vi "Eval LTFC.vi"(8 "error in (no error)":errorcluster, 10 "Desired Field (T)":dbl) -> (0 "error out":errorcluster, 2 "Desired Control Voltage":dbl)   [LabVIEW 2009, in "Varian Magnet.lvclass"]
doc: "Evaluates Long-Term Field Calibration for control voltage that corresponds to desired field.\nAlso error checks to see if Long-Term Field Calibration is initialized properly."
uses:
  Varian Magnet.lvclass
  Varian Constants.vi
  <vilib>/Utility/error.llb/DialogType.ctl
  <vilib>/gmath/NI_Gmath.lvlib
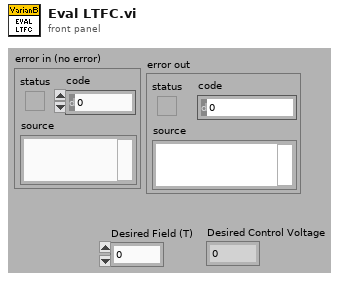
[diagram p1: front panel]
types:
  T1 = typedef "NI_Gmath.lvlib/in_piecewise interp poly control.ctl" = cluster{"x locations":dbl[], "coefficients":dbl[][]}
  T2 = typedef "DialogType.ctl" = u16
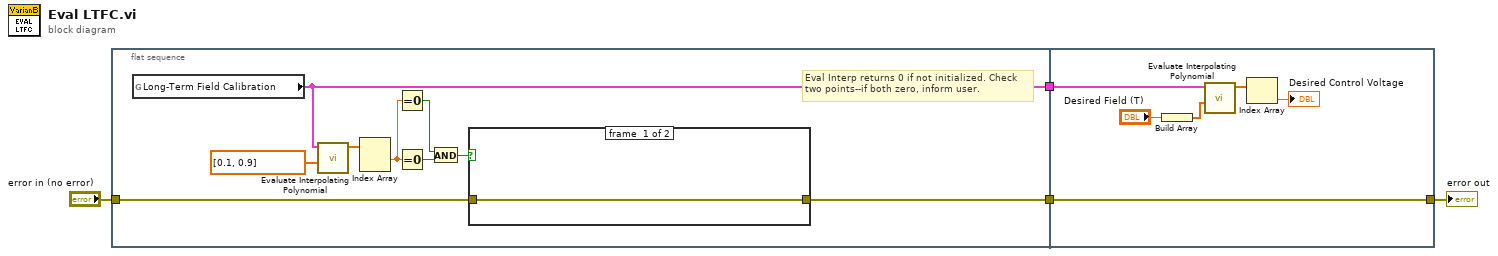
[diagram p0: block diagram]
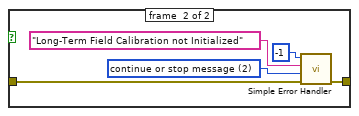
[diagram p2: hidden frame]
diagram:
  n1 = flat-sequence {
    tunnel: "error in (no error)" -> [w7]
    tunnel: [w6] -> w3
    tunnel: [w5] -> w2
    tunnel: [w25] -> w1
    tunnel: w3 -> [w25]
    tunnel: w2 -> [w23]
    frame #0 {
      # "Eval Interp returns 0 if not initialized. Check\ntwo points--if both zero, inform user."
      n2 = global read "Varian Constants.vi" "Long-Term Field Calibration"() -> (w5:T1)
      n3 = call <vilib>:"Evaluate Interpolating Polynomial.vi"("xi"=dbl[] [0.1, 0.9], "piecewise polynomial"=w5) -> ("yi"=w13:dbl[])  [unwired: 8 in, 1 out]
      n4 = Index Array(array=w13) -> (element #1=w11:dbl)  [unwired: 2 in, 1 out]
      n5 = Equal To 0?(x=w11) -> (x = 0?=w10:bool)
      n6 = Equal To 0?(x=w11) -> (x = 0?=w9:bool)
      n7 = And(x=w10, y=w9) -> (x .and. y?=w8:bool)
      n8 = case shown="True" w8 {
        tunnel: w7 -> [w14 w16]
        tunnel: [w14 w15] -> w6
        frame #0 {
        }
        frame #1 {
          w17 = T2 2 items=["no dialog", "OK message", "continue or stop message", "OK message + warnings", "continue/stop + warnings"] ("type of dialog (OK msg:1)")
          n9 = call <vilib>:"Simple Error Handler.vi"("error code (no error:0)"=-1, "error source (\" \")"="Long-Term Field Calibration not Initialized" ("error source (\" \")"), "type of dialog (OK msg:1)"=w17, "error in (no error)"=w16) -> ("error out"=w15:errorcluster)  [unwired: 1 in, 4 out]
        }
      }
    }
    frame #1 {
      n10 = Build Array("Desired Field (T)") -> (w21:dbl[])
      n11 = call <vilib>:"Evaluate Interpolating Polynomial.vi"("xi"=w21, "piecewise polynomial"=w23) -> ("yi"=w24:dbl[])  [unwired: 8 in, 1 out]
      n12 = Index Array(array=w24) -> (element=→"Desired Control Voltage":dbl)  [unwired: 1 in]
    }
  }
  "error out" <- w1
